vi "DataStream_RTQ_Create.vi"(11 "Close Queue":bool) -> (3 "RTQ":refnum<queue>)   [LabVIEW 2020]
uses:
  TypeDefs/Cluster_DataStream RT Data Set.ctl
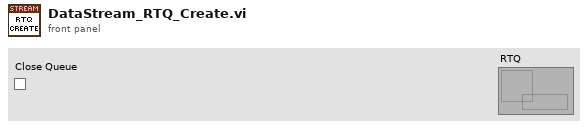
[diagram p1: front panel]
types:
  T1 = typedef "Cluster_DataStream RT Data Set.ctl" = cluster{"Header Array":string[], "Time Stamp Array":dbl[], "Value Array":dbl[]}
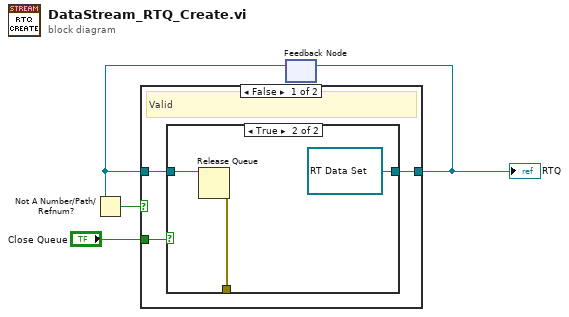
[diagram p0: block diagram]
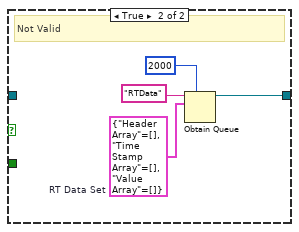
[diagram p3: hidden frame]
diagram:
  n1 = feedback #1() -> (w2:refnum<queue>)  [unwired: 1 in]
  n2 = Not A Number/Path/Refnum?(number/path/refnum=w2) -> (NaN/Path/Refnum?=w3:bool)
  n3 = case shown="False" w3 {
    tunnel: [w5 w13] -> w4
    tunnel: w2 -> [w6 _]
    tunnel: "Close Queue" -> [w7 _]
    frame False {
      # "Valid"
      n4 = case shown="True" w7 {
        tunnel: w6 -> [w8 w11]
        tunnel: [w8 refnum<queue> refnum ("queue out")] -> w5
        tunnel: [_ w10] -> _
        frame False {
        }
        frame True {
          n5 = Release Queue(queue=w11) -> (error out=w10:errorcluster)  [unwired: 2 in, 2 out]
        }
      }
    }
    frame True {
      w15 = T1 {"Header Array"=[], "Time Stamp Array"=[], "Value Array"=[]}  # RT Data Set
      # "Not Valid"
      n6 = Obtain Queue(max queue size (-1, unlimited)=2000, name (unnamed)="RTData", element data type=w15) -> (queue out=w13:refnum<queue>)  [unwired: 2 in, 2 out]
    }
  }
  "RTQ" <- w4
  n7 = feedback-in #1(w4) -> ()
